vi "雷达流速仪写数据库.vi"(8 "错误输入（无错误）":errorcluster, 11 "采集数据":T2) -> (0 "错误输出":errorcluster)   [LabVIEW 2016, in "雷达流速仪.lvlib"]
panel:
  in  "仪器":string="雷达流速仪"
  in  "data":T1
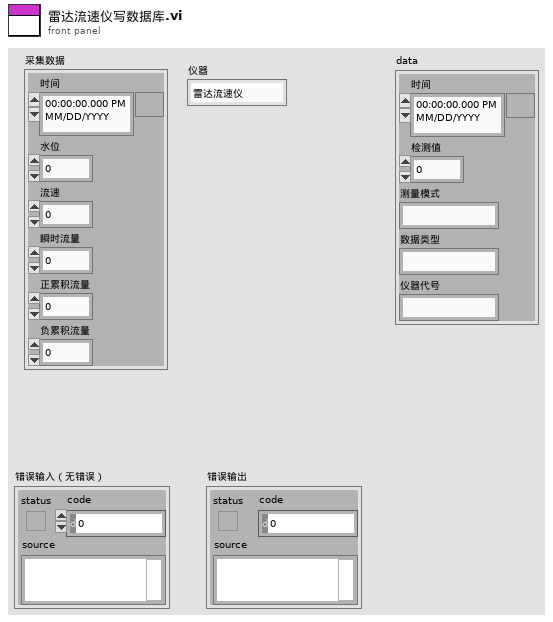
[diagram p1: front panel]
types:
  T1 = cluster{"时间":timestamp, "检测值":dbl, "测量模式":string, "数据类型":string, "仪器代号":string}
  T2 = cluster{"时间":timestamp, "水位":dbl, "流速":dbl, "瞬时流量":dbl, "正累积流量":dbl, "负累积流量":dbl}
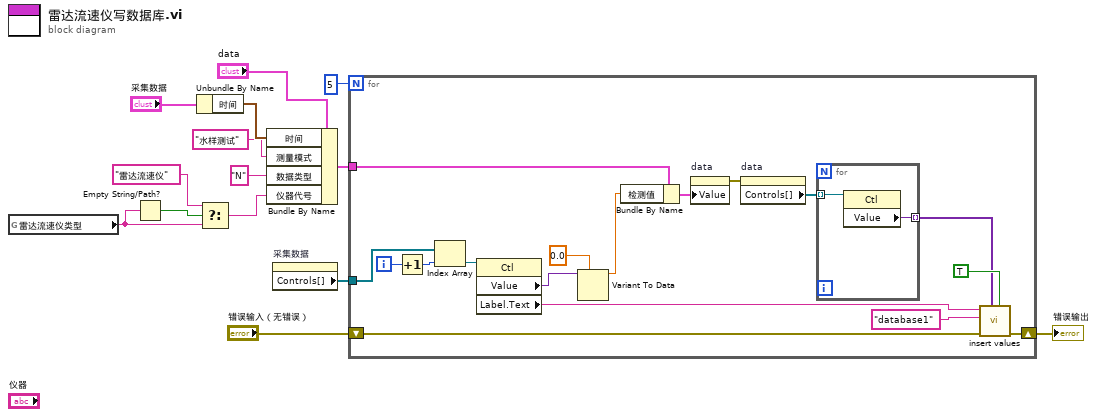
[diagram p0: block diagram]
diagram:
  n1 = global read "雷达流速仪全局变量.vi" "雷达流速仪类型"() -> (w2:string)
  n2 = Empty String/Path?(string/path=w2) -> (empty?=w4:bool)
  n3 = Unbundle By Name("采集数据") -> ("时间"=w12:timestamp)
  n4 = Select(t="雷达流速仪", s=w4, f=w2) -> (s? t:f=w1:string)
  n5 = Bundle By Name(cluster="data", "时间"=w12, "测量模式"="水样测试", "数据类型"="N", "仪器代号"=w1) -> (w8:T1)
  n6 = property on="采集数据" class="Clust (strict)"() -> ("Controls[]"=w7:refnum<vi>[])  [unwired: 2 in, 2 out]
  n7 = for {
    N: 5 -> [_]
    tunnel: w8 -> [w24]
    tunnel: w7 -> [w30]
    shift-right: [w16] -> w5
    shift-left: "错误输入（无错误）" -> [w17]
    i -> [w31]
    n8 = Increment(x=w31) -> (x+1=w29:i32)
    n9 = Index Array(array=w30, index=w29) -> (element=w28:refnum<vi>)
    n10 = property class="Ctl"(reference=w28) -> ("Value"=w25:variant, "Label.Text"=w15:string)  [unwired: 1 in, 2 out]
    n11 = Variant To Data(type=0.0, Variant=w25) -> (data=w27:dbl)  [unwired: 1 in, 1 out]
    n12 = Bundle By Name(cluster=w24, "检测值"=w27) -> (w23:T1)
    n13 = property on="data" class="Clust (strict)"("Value"=w23) -> (error out=w22:errorcluster)  [unwired: 2 in, 1 out]
    n14 = property on="data" class="Clust (strict)"(error in=w22) -> ("Controls[]"=w18:refnum<vi>[])  [unwired: 1 in, 2 out]
    n15 = for {
      tunnel: w18 -> [w33] mode=indexing
      tunnel: [w32] -> w19 mode=indexing
      n16 = property class="Ctl"(reference=w33) -> ("Value"=w32:variant)  [unwired: 1 in, 2 out]
    }
    n17 = call "insert values.vi"("是否创建唯一键"=TRUE, "data"=w19, "错误输入（无错误）"=w17, "database"="database1", "Tabe Name"=w15) -> ("错误输出"=w16:errorcluster)  [unwired: 6 in]
  }
  "错误输出" <- w5
